vi "Motion_xbee_2Radars.vi"(0 "VISA resource name":refnum<visa-resource-name>="COM1", 1 "baud rate":u32=9600, 4 "data bits":u16=8 min=5 max=8 step=1, 5 "parity":u16(ring) items=["None", "Odd", "Even", "Mark", "Space"], 7 "stop bits":u16=10, 9 "XON Character":u8=17 format="%.0x", 14 "XOFF Character":u8=19 format="%.0x", 15 "timeout (ms)":u32=10000, 21 "End read on termination character?":bool, 24 "termination char\n(0xA = '\\n' = LF)":u8=10 format="%.0x", 25 "buffer size":u32=4096) -> ()   [LabVIEW 2015]
doc: "The Advanced Serial Read and Write example performs a Serial Port Read, a Serial Port Write, or a combination of these actions while setting some advanced serial features like buffer size, termination characters, and XON/XOFF flow control. The user selects the actions (read or write) on the front panel. If both are selected, the VI will write the data first, read the data and then close the VISA session that is opened to the port. \n\nThe parameters set for the serial port must match the parameters of the connected instrument or device. In this example, the bytes to read parameter specifies the number of bytes that the serial port reads. If there were more bytes at the port than the number specified in bytes to read, those bytes would not be read. Also, if you specify to read more bytes than the number of bytes actually read, you might receive a timeout error message.\n\nINSTRUCTIONS:\n1) Select the serial resource and configuration parameters (baud rate, data bits, parity, stop bits, flow control).\n2) Termination character can be enabled and set. Also, set the required input buffer size prior to running the example.\n3) Select the operations to be performed. \n4) Connect the serial port to your device. If no device is available, perform a loopback test by doing one of the following. Short pins 2 and 3 on a RS-232 cable or short pin 4 to pin 8 and pin 5 to pin 9 on a RS-485/422 cable. \n5) Run the VI to see the data read. (The \"read string\" will match the \"string to write\" if a loopback test was performed.)\n\nThis example exposes several advanced features that you may need for your application. Not all applications need all the features shown in this example. The input buffer size is likely an important setting that you want to control in your application. This example expands upon the flow control option for XON and XOFF, allowing the user to choose those control characters. The timeout parameter has been brought to the front panel so a user can specify the time period the VISA Read will wait for the number of bytes to read before timing out. Also, the user has several controls for the termination character, which is discussed later.\n\nNote that you can press the write and read buttons and change the bytes to read parameters on the fly, while the example is running. However, you must stop the example to change the other configuration parameters after the example has started running, and then run again.\n\nSet the I/O buffer size slightly higher the amount of data you expect to receive. This is very important for applications that don't use flow control, as you may lose characters if the receive buffer overflows.\n\nSetting the timeout period ensures that the operation returns with a timeout error if the operation cannot be performed in the specified time period. \n\nSome devices require a termination character in order to identify the end of command strings. Some devices send a termination character to signify the end of data to be read. \n\nThis example shows how you can end the Read operation once a termination character is detected in the buffer and/or append a termination character at the end of the Write data. To enable the Read to end on a termination character, use the VISA Configure Serial Port or use the VISA Properties Serial End Mode for Reads, Termination Character Enable, and Termination Character. To end the Write with a termination character, use the VISA Properties Serial End Mode for Writes, the Send End Enable, and Termination Character. In this example, the same termination character is used for both the Read and the Write. You can specify two different characters for your application, if desired.\n\nYour application may require specific characters for the XON/XOFF Flow Control. You can specify these characters with the VISA Properties Flow Control XOFF Character and Flow Control XON Character. Note that if the standard XON and XOFF characters are used, then decimal 17 and 19 are unavailable for data values. Remember that using flow control and setting an adequate buffer size allow you to prevent buffer overflows."
uses:
  <vilib>/Instr/_visa.llb/VISA Configure Serial Port (Instr).vi
panel:
  out "I/Q channels 2":dynamicdata(graph)
  out "Spectrum 2":waveform(dbl)(graph)
  out "Spectrum":waveform(dbl)(graph)
  out "I/Q channels":dynamicdata(graph)
  in  "Data saving path":path=path "C:/Users/zpeng/OneDrive - Texas Tech University/Desktop/BeamSteering/data"
  in  "Save raw data":bool
  in  "FFT":i32=256
  in  "flow control":u16(ring) items=["None"=0, "XON/XOFF"=1, "RTS/CTS"=2, "DTR/DSR"=4]
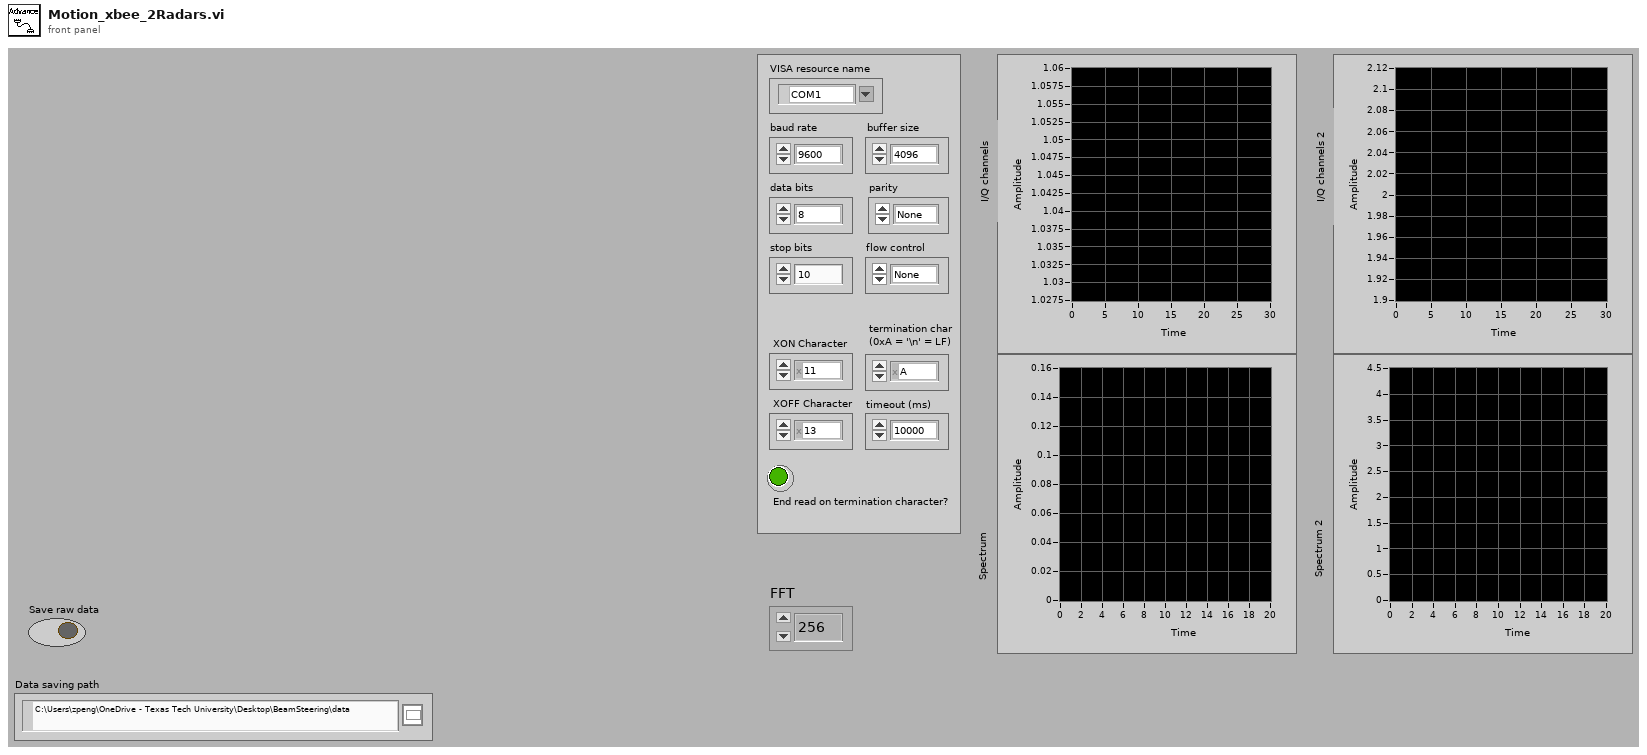
[diagram p1: front panel]
types:
  T1 = cluster{"VISA resource name out":refnum<visa-resource-name>, "error IO":errorcluster, "y":u8, i32, "Data saving path":path, "Save raw data":bool}
  T2 = cluster{"VISA resource out ":refnum<visa-resource-name>, "error out":errorcluster, "y":u8, i32, "Data saving path":path, "Save raw data":bool}
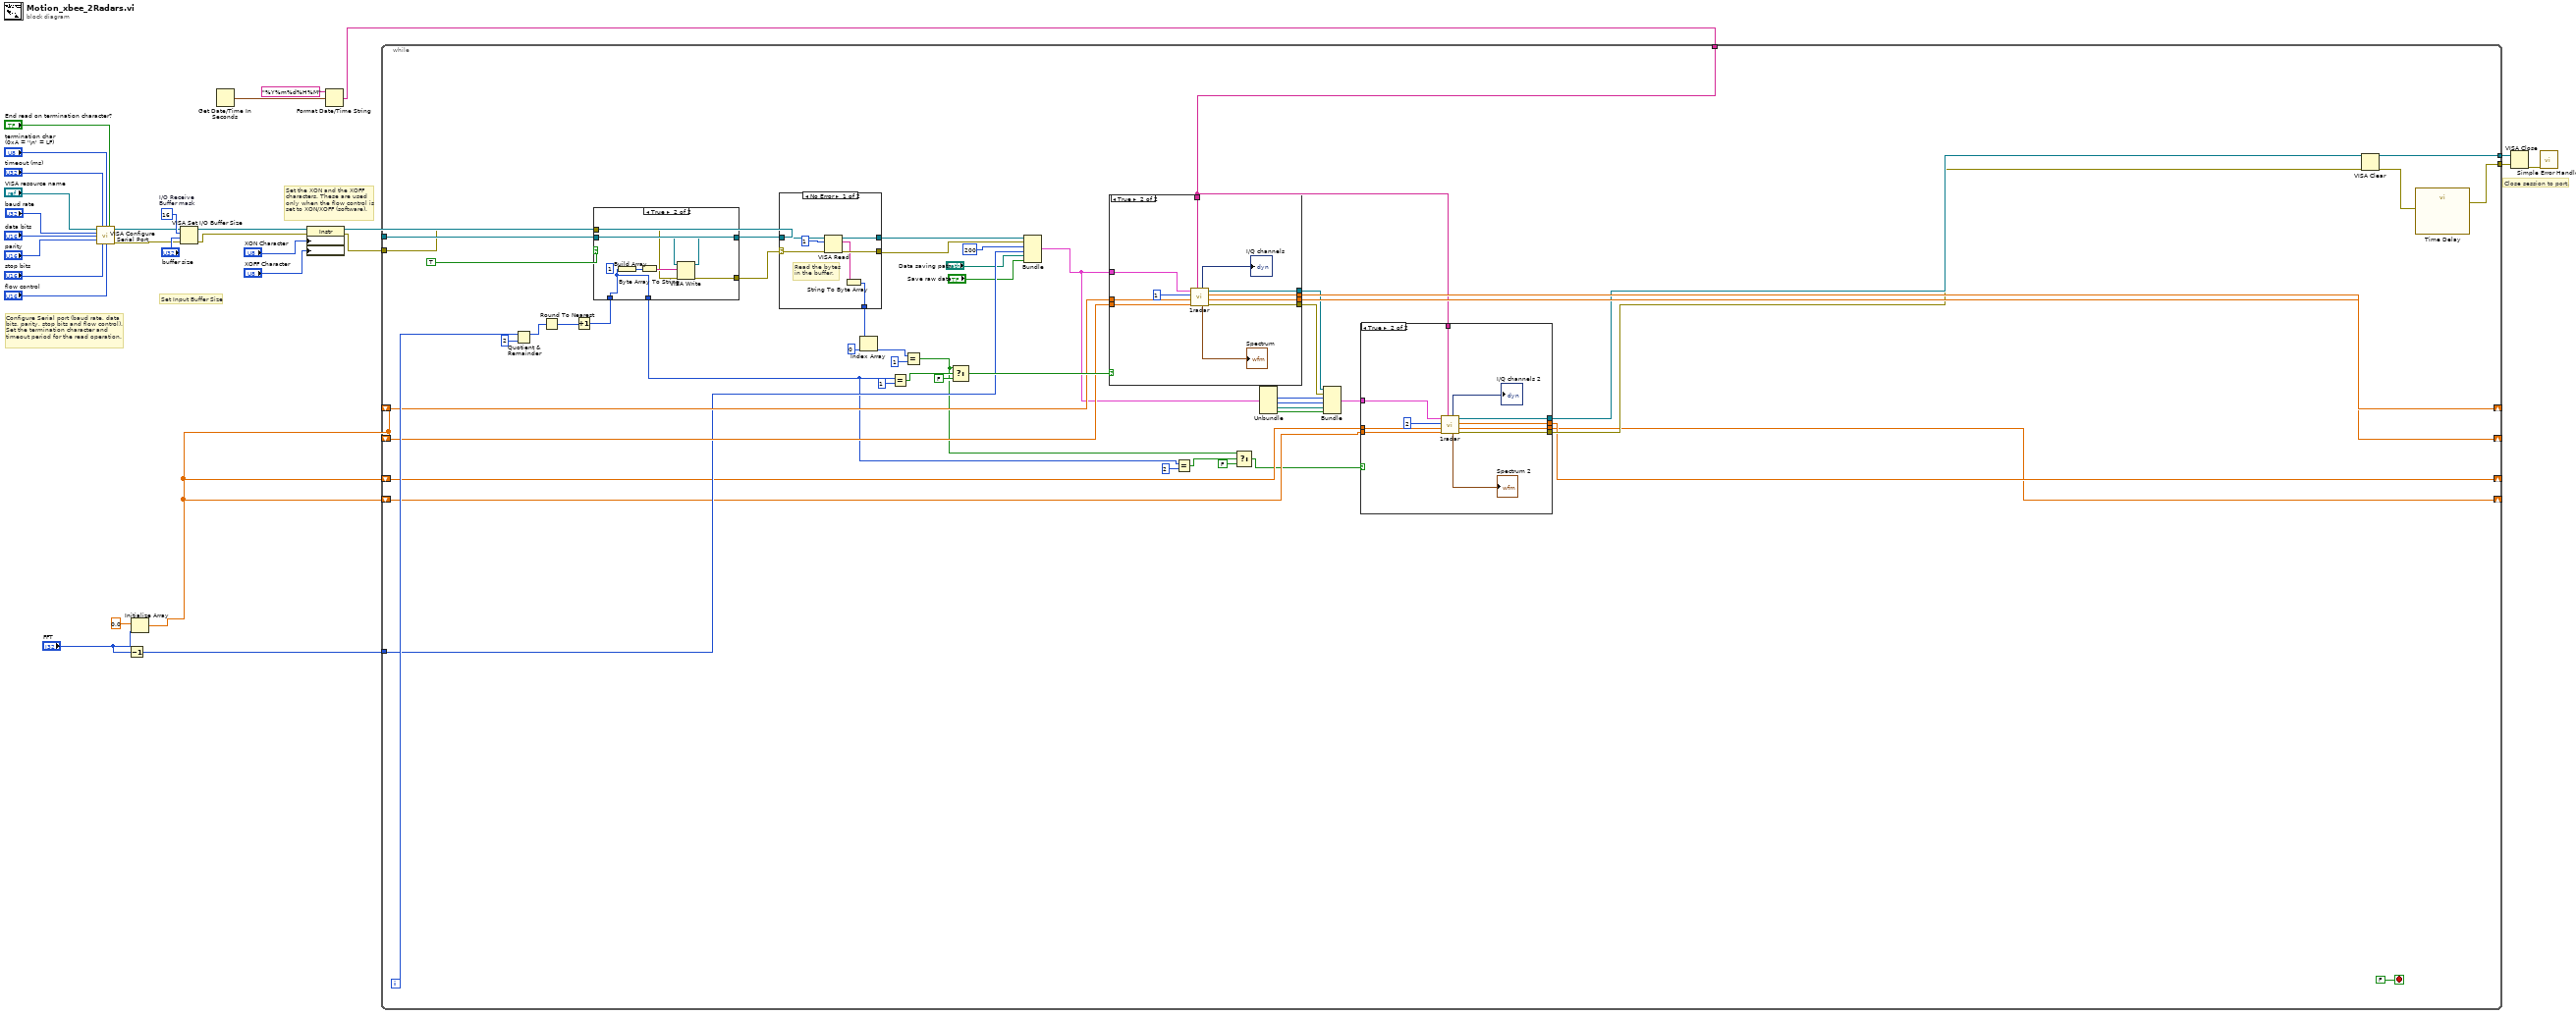
[diagram p0: block diagram]
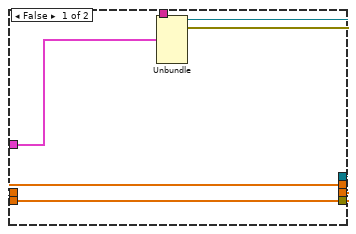
[diagram p2: hidden frame]
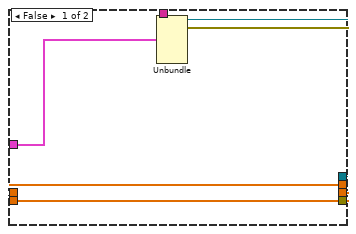
[diagram p4: hidden frame]
diagram:
  w22 = u16 16  # I/O Receive Buffer mask
  # "Set the XON and the XOFF\ncharacters. These are used\nonly when the flow control is\nset to XON/XOFF (software)."
  # "Configure Serial port (baud rate, data\nbits, parity, stop bits and flow control).\nSet the termination character and\ntimeout period for the read operation."
  # "Set Input Buffer Size"
  # "Close session to port."
  n1 = call-poly "VISA Configure Serial Port"("VISA resource name"="VISA resource name", "timeout (10sec)"="timeout (ms)", "termination char\n(0xA = '\\n' = LF)"="termination char\n(0xA = '\\n' = LF)", "Enable Termination\nChar (T)"="End read on termination character?", "baud rate (9600)"="baud rate", "data bits (8)"="data bits", "parity (0:none)"="parity", "stop bits (10: 1 bit)"="stop bits", "flow control (0:none)"="flow control") -> ("VISA resource name out"=w8:refnum<visa-resource-name>, "error out"=w7:errorcluster)  [unwired: 1 in, 4 out]
  n2 = Decrement(x="FFT") -> (x-1=w11:i32)
  n3 = Initialize Array(0.0 ("element"), "FFT") -> (w1:dbl[])
  n4 = VISA Set I/O Buffer Size(VISA resource name=w8, mask (16)=w22, size (4096)="buffer size", error in (no error)=w7) -> (VISA resource name out=w18:refnum<visa-resource-name>, error out=w17:errorcluster)
  n5 = Get Date/Time In Seconds() -> (seconds since 1Jan1904=w3:timestamp)
  n6 = property class="Instr"(reference=w18, error in=w17, "Serial Settings:Flow Control XON Character"="XON Character", "Serial Settings:Flow Control XOFF Character"="XOFF Character") -> (reference out=w6:refnum<visa-resource-name>, error out=w5:errorcluster)
  n7 = Format Date/Time String(time format string (%c)="%Y%m%d%H%M", seconds (now)=w3) -> (date/time string=w2:string)  [unwired: 1 in]
  n8 = while {
    tunnel: w11 -> [w53]
    tunnel: w6 -> [w78]
    tunnel: [w74] -> w13
    tunnel: w5 -> [w79]
    tunnel: [w76] -> w12
    shift-right: [w80] -> _
    shift-left: w1 -> [w57]
    shift-right: [w81] -> _
    shift-left: w1 -> [w58]
    tunnel: w2 -> [w38]
    shift-right: [w37] -> _
    shift-left: w1 -> [w44]
    shift-right: [w36] -> _
    shift-left: w1 -> [w43]
    i -> [w67]
    stop <- FALSE stop-if-true
    n9 = Quotient & Remainder(x=w67, y=2) -> (x-y*floor(x/y)=w68:i32)  [unwired: 1 out]
    n10 = Round To Nearest(number=w68) -> (nearest integer value=w65:i32)
    n11 = Increment(x=w65) -> (x+1=w62:i32)
    n12 = case shown="True" TRUE {
      tunnel: w79 -> [w126 w132]
      tunnel: w78 -> [w125 w131]
      tunnel: [w125 w130] -> w72
      tunnel: [w126 w129] -> w73
      tunnel: w62 -> [_ w127]
      tunnel: [_ w127] -> w31
      frame False {
      }
      frame True {
        (unwired) u8 1 ("element")
        n13 = Build Array(w127) -> (w128:i32[])
        n14 = Byte Array To String(unsigned byte array=w128) -> (string=w133:string)
        n15 = VISA Write(VISA resource name=w131, write buffer=w133, error in (no error)=w132) -> (VISA resource name out=w130:refnum<visa-resource-name>, error out=w129:errorcluster)  [unwired: 1 out]
      }
    }
    n16 = case "Read bytes from port." shown="No Error" w73 {
      selector: w73 -> [w102 w107]
      tunnel: [w104 w107] -> w55
      tunnel: [w105 w108] -> w56
      tunnel: w72 -> [w103 w108]
      tunnel: [w100 u8[] [] ("unsigned byte array")] -> w71
      frame No Error {
        # "Read the bytes\nin the buffer."
        n17 = VISA Read(VISA resource name=w103, byte count=u32 1, error in (no error)=w102) -> (VISA resource name out=w105:refnum<visa-resource-name>, read buffer=w101:string, error out=w104:errorcluster)  [unwired: 1 out]
        n18 = String To Byte Array(string=w101) -> (unsigned byte array=w100:u8[])
      }
      frame Error {
        # "Error occurred \nreading Bytes at \nSerial Port"
      }
    }
    n19 = Index Array(array=w71, index=0) -> (element=w69:u8)
    n20 = Equal?(x=w31, y=1) -> (x = y?=w60:bool)
    n21 = Equal?(x=w69, y=u8 1) -> (x = y?=w32:bool)
    n22 = Select(t=w32, s=w60, f=FALSE) -> (s? t:f=w64:bool)
    n23 = Bundle("VISA resource name out"=w56, "error IO"=w55, "y"=u8 200, w53, "Data saving path"="Data saving path", "Save raw data"="Save raw data") -> (w50:T1)  [unwired: 1 in]
    n24 = case shown="True" w64 {
      tunnel: [w113 w118] -> w81
      tunnel: [w112 w117] -> w80
      tunnel: [w110 w120] -> w42
      tunnel: [w109 w119] -> w40
      tunnel: w38 -> [_ w116]
      tunnel: w58 -> [w113 w122]
      tunnel: w57 -> [w112 w121]
      tunnel: w50 -> [w111 w124]
      frame False {
        n25 = Unbundle(w111) -> ("VISA resource name out"=w110:refnum<visa-resource-name>, "error IO"=w109:errorcluster)  [unwired: 4 out]
      }
      frame True {
        n26 = call "1radar.vi"("date/time string"=w116, "Q"=w121, "I"=w122, "radar number"=u8 1 ("y"), "input cluster"=w124) -> ("error out"=w119:errorcluster, "Q out"=w117:dbl[], "I out"=w118:dbl[], "VISA resource out"=w120:refnum<visa-resource-name>, "Spectrum"=→"Spectrum":waveform(dbl), "I/Q channels"=→"I/Q channels":dynamicdata)  [unwired: 1 in]
      }
    }
    n27 = Equal?(x=w31, y=2) -> (x = y?=w35:bool)
    n28 = Select(t=w32, s=w35, f=FALSE) -> (s? t:f=w30:bool)
    n29 = Unbundle(w50) -> ("y"=w49:u8, w48:i32, "Data saving path"=w47:path, "Save raw data"=w46:bool)  [unwired: 2 out]
    n30 = Bundle("VISA resource out"=w42, "error out"=w40, "y"=w49, w48, "Data saving path"=w47, "Save raw data"=w46) -> (w45:T2)  [unwired: 1 in]
    n31 = case shown="True" w30 {
      tunnel: [w87 w92] -> w37
      tunnel: [w86 w91] -> w36
      tunnel: [w84 w94] -> w41
      tunnel: [w83 w93] -> w39
      tunnel: w38 -> [_ w90]
      tunnel: w44 -> [w87 w96]
      tunnel: w43 -> [w86 w95]
      tunnel: w45 -> [w85 w98]
      frame False {
        n32 = Unbundle(w85) -> ("VISA resource out"=w84:refnum<visa-resource-name>, "error out"=w83:errorcluster)  [unwired: 4 out]
      }
      frame True {
        n33 = call "1radar.vi"("date/time string"=w90, "Q"=w95, "I"=w96, "radar number"=u8 2 ("y"), "input cluster"=w98) -> ("error out"=w93:errorcluster, "Q out"=w91:dbl[], "I out"=w92:dbl[], "VISA resource out"=w94:refnum<visa-resource-name>, "Spectrum"=→"Spectrum 2":waveform(dbl), "I/Q channels"=→"I/Q channels 2":dynamicdata)  [unwired: 1 in]
      }
    }
    n34 = VISA Clear(VISA resource name=w41, error in (no error)=w39) -> (VISA resource name out=w74:refnum<visa-resource-name>, error out=w75:errorcluster)
    n35 = call "Time Delay"("error in (no error)"=w75) -> ("error out"=w76:errorcluster)  [unwired: 10 in]
  }
  n36 = VISA Close(VISA resource name=w13, error in (no error)=w12) -> (error out=w27:errorcluster)
  n37 = call <vilib>:"Simple Error Handler.vi"("error in (no error)"=w27) -> ()  [unwired: 1 in, 8 out]
